vi "Constants.vi"() -> ()   [LabVIEW 2015, in "Modbus Master Shared.lvlib"]
doc: "Use this Global VI to access the GUIDs assigned to the page resources of the Custom Device."
uses:
  Modbus Master Shared.lvlib
panel:
  in  "Tab Control":T1(tab)=enum."Interface Properties"
  in  "Ex5":string="9528fbce-cba9-4b33-ba5b-9ac98a79e3e4"
  in  "Ex4":string="817ae295-493c-4301-8e84-eaa9bb3bfa8f"
  in  "Ex3":string="3058d819-b633-4a2e-8348-09d520a4405b"
  in  "Diagnostics Group":string="df02c6b5-4e9c-4d13-ab55-0b56edc10372"
  in  "Error Group":string="602ecb33-008e-4c4e-a9be-75d53d19e154"
  in  "AO Reg UI":string="a01a3473-157c-4b35-9b7d-138555919c7d"
  in  "AI Reg UI":string="0c4b7bf5-0426-4a85-9a56-9146af84f771"
  in  "DO Coil UI":string="b31ca022-9f15-479b-8121-bb367a79ccc6"
  in  "DI Coil UI":string="80038b18-1d4d-4c59-bd93-ea1908a5e402"
  in  "AO Regs Group UI":string="084ec162-0c92-47f2-8a13-adc6b3468b40"
  in  "AI Regs Group UI":string="7b1a17fc-6305-41c5-ad32-5ce3c3895b98"
  in  "DO Coils Group UI":string="e1d5ecdc-886d-4452-883e-444ae499dbea"
  in  "DI Coils Group UI":string="6b758301-dafc-4492-9cfa-219aa899e425"
  in  "Interface UI":string="0a20a8c5-366f-406e-8864-c24e8e6076a5"
  in  "Modbus Master":string="1199cc90-62ea-4be2-b123-96c31660e707"
  in  "Group.Outgoing.HoldingRegisters":string="Group Outgoing Holding Registers"
  in  "Group.Outgoing.Coils":string="Group Outgoing Coils"
  in  "Group.Incoming.InputRegisters":string="Group Incoming Input Registers"
  in  "Group.Incoming.DiscreteInputs":string="Group Incoming Discrete Inputs"
  in  "Runtime.Settings":string="Runtime Settings"
  in  "Interface.TCP.Timeout":string="Interface TCP Timeout"
  in  "Interface.MaxGroupSize":string="Interface Max Group Size"
  in  "Interface.Timeout?":string="Interface Timeout"
  in  "Interface.LateReadCount":string="Interface Late Read Count"
  in  "Interface.RefreshRate":string="Interface Refresh Rate"
  in  "Interface.Alias":string="Interface Alias"
  in  "Interface.Serial.FlowControl":string="Interface Serial Flow Control"
  in  "Interface.Serial.WireMode":string="Interface Serial Wire Mode"
  in  "Interface.Serial.Type":string="Interface Serial Type"
  in  "Interface.Serial.Parity":string="Interface Serial Parity"
  in  "Interface.Serial.BaudRate":string="Interface Serial Baud Rate"
  in  "Interface.Serial.VISAResourceName":string="Interface Serial VISA Resource Name"
  in  "Interface.TCP.Port":string="Interface TCP Port"
  in  "Interface.TCP.Address":string="Interface TCP Address"
  in  "Interface.UnitID":string="Interface Unit ID"
  in  "Interface.Type":string="Interface Type"
  in  "Coil.Direction":string="Coil Direction"
  in  "Coil.StartingAddress":string="Coil Starting Address"
  in  "Input Register.Direction":string="Input Register Direction"
  in  "InputRegister.DataType":string="Input Register Data Type"
  in  "InputRegister.SubAddress":string="Input Register Sub Address"
  in  "InputRegister.StartingAddress":string="Input Register Starting Address"
  in  "Discrete Input.Direction":string="Discrete Input Direction"
  in  "DiscreteInput.StartingAddress":string="Discrete Input Starting Address"
  in  "Holding Register.Direction":string="Holding Register Direction"
  in  "HoldingRegister.DataType":string="Holding Register Data Type"
  in  "HoldingRegister.SubAddress":string="Holding Register Sub Address"
  in  "HoldingRegister.Starting Address":string="Holding Register Starting Address"
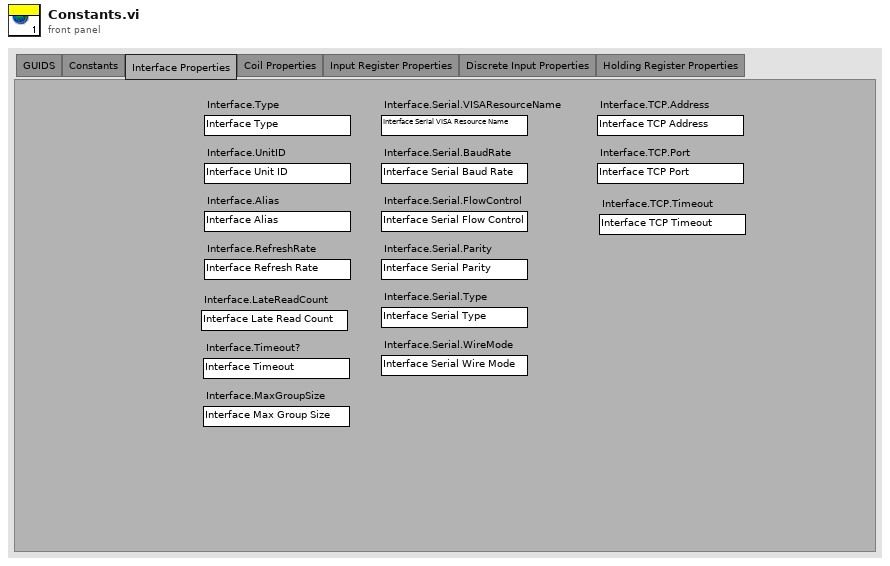
[diagram p1: front panel]
types:
  T1 = enum32{"GUIDS", "Constants", "Interface Properties", "Coil Properties", "Input Register Properties", "Discrete Input Properties", "Holding Register Properties"}
diagram:
